vi "tituloDoArquivo.vi"(6 "area":i64 caption="Área da célula", 7 "irradiancia":dbl, 8 "temperatura":i64 caption="Temperatura da célula", 9 "Tipo":string caption="Tipo da célula", 10 "Nome da célula":string, 11 "file path (dialog if empty)":path) -> ()   [LabVIEW 2012]
uses:
  <vilib>/Utility/file.llb/Write To Spreadsheet File (string).vi
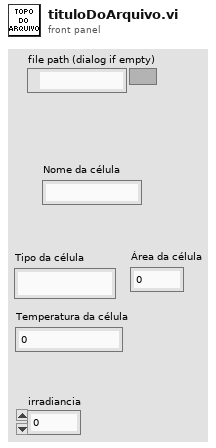
[diagram p1: front panel]
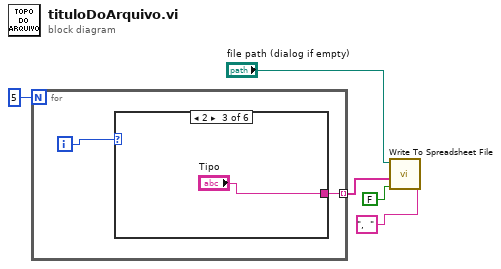
[diagram p0: block diagram]
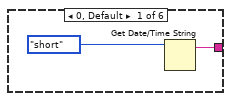
[diagram p2: hidden frame]
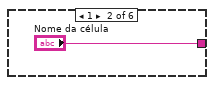
[diagram p3: hidden frame]
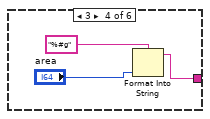
[diagram p4: hidden frame]
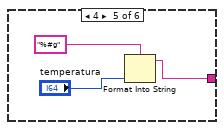
[diagram p5: hidden frame]
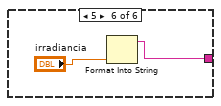
[diagram p6: hidden frame]
diagram:
  n1 = for {
    N: 5 -> [_]
    tunnel: [w7] -> w5 mode=indexing
    i -> [w6]
    n2 = case shown="2" w6 {
      tunnel: [w9 "Nome da célula" "Tipo" w13 w16 w19] -> w7
      frame 0, Default {
        n3 = Get Date/Time String(date format (0)=enum16{"short", "long", "abbreviated"}."short") -> (date string=w9:string)  [unwired: 2 in, 1 out]
      }
      frame 1 {
      }
      frame 2 {
      }
      frame 3 {
        n4 = Format Into String(format string="%#g", "area") -> (resulting string=w13:string)  [unwired: 2 in, 1 out]
      }
      frame 4 {
        n5 = Format Into String(format string="%#g", "temperatura") -> (resulting string=w16:string)  [unwired: 2 in, 1 out]
      }
      frame 5 {
        n6 = Format Into String("irradiancia") -> (resulting string=w19:string)  [unwired: 3 in, 1 out]
      }
    }
  }
  n7 = call-poly <vilib>:"Write To Spreadsheet File.vi"("delimiter (\\t)"=",  " ("delimiter (\\t)"), "append to file? (new file:F)"=FALSE, "1D data"=w5, "file path (dialog if empty)"="file path (dialog if empty)") -> ()  [unwired: 4 in, 1 out]
